vi "AlliGator Update Channel File Settings.vi"(8 "Error In":errorcluster, 9 "Channel Arithmetic":T1, 10 "Selected Channel Name":string, 11 "Available Channel Names":string[](array[string])) -> (0 "Error Out":errorcluster)   [LabVIEW 2021, in "AlliGator Settings.lvlib"]
doc: "Updates the values of the <B>Channel Name</b> and <B>Channel Arithmetic</b> controls, as well as of the hidden <B>Available Channel Names</b> indicator."
uses:
  AlliGator Settings.lvlib
  AlliGator Gate Arithmetic.ctl
  AlliGator Settings Event.ctl
  AlliGator Settings Window Messages.ctl
  AlliGator Dual-Channel Datasets.lvlib
panel:
  # "see the AlliGator License on the block diagram (Ctrl+E or Window:Show Block Diagram)"
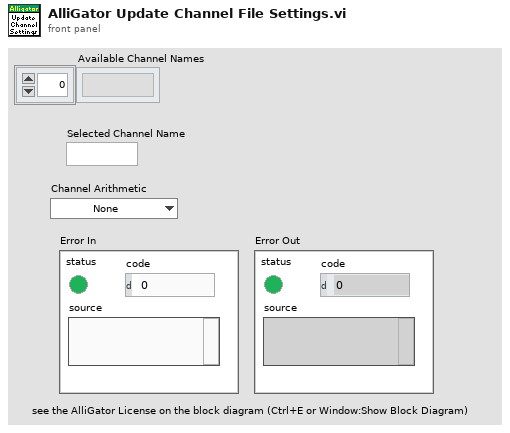
[diagram p1: front panel]
types:
  T1 = typedef "AlliGator Settings.lvlib/AlliGator Gate Arithmetic.ctl" = enum16{"None", "INT-G2", "G2/INT*<INT>", "(1 - G2/INT)*<INT>"}
  T2 = typedef "AlliGator Settings.lvlib/AlliGator Settings Event.ctl" = cluster{"AlliGator Settings Message":T3, "Sender":string, "Control Label":string, "Data":variant}
  T3 = typedef "AlliGator Settings.lvlib/AlliGator Settings Window Messages.ctl" = enum16{"Idle", "Subscribe", "Unsubscribe", "Refresh Parameter", "Refresh All Parameters", "Quit"}
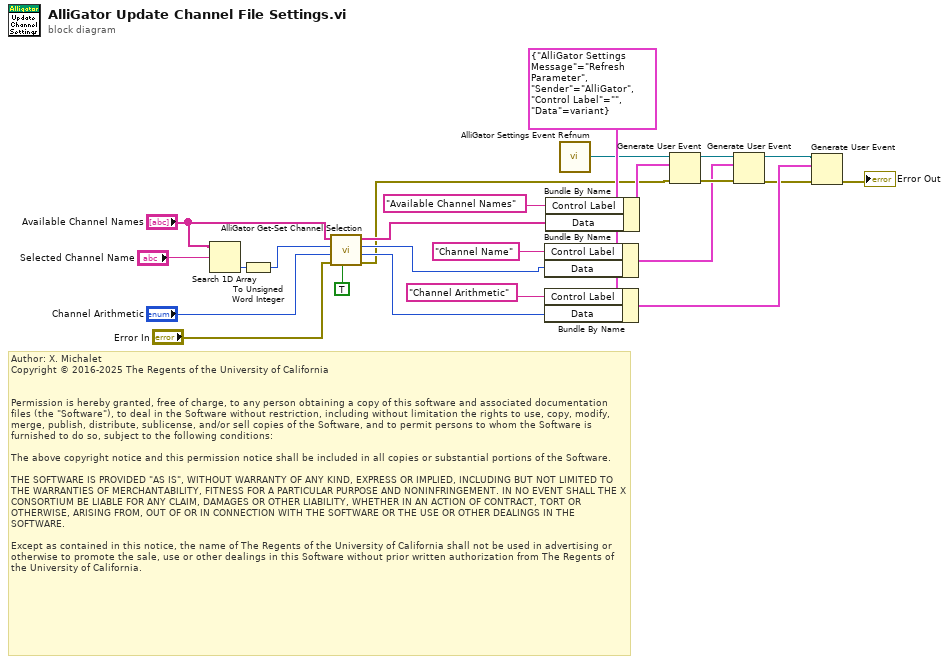
[diagram p0: block diagram]
diagram:
  w18 = T2 {"AlliGator Settings Message"=enum."Refresh Parameter", "Sender"="AlliGator", "Control Label"="", "Data"=variant} ("event data")
  # "Author: X. Michalet\nCopyright © 2016-2025 The Regents of the University of California\n \n\nPermission is hereby granted, free of charge, to any person obtaining a copy of this software and associated documentation files (the \"Software\"), to deal in the Software without restriction, including without limitation the rights to use, copy, modify, merge, publish, distribute, sublicense, and/or sell copies of the Software, and to permit persons to whom the Software is furnished to do so, subject to the following conditions:\n\nThe above copyright notice and this permission notice shall be included in all copies or substantial portions of the Software.\n\nTHE SOFTWARE IS PROVIDED \"AS IS\", WITHOUT WARRANTY OF ANY KIND, EXPRESS OR IMPLIED, INCLUDING BUT NOT LIMITED TO THE WARRANTIES OF MERCHANTABILITY, FITNESS FOR A PARTICULAR PURPOSE AND NONINFRINGEMENT. IN NO EVENT SHALL THE X CONSORTIUM BE LIABLE FOR ANY CLAIM, DAMAGES OR OTHER LIABILITY, WHETHER IN AN ACTION OF CONTRACT, TORT OR OTHERWISE, ARISING FROM, OUT OF OR IN CONNECTION WITH THE SOFTWARE OR THE USE OR OTHER DEALINGS IN THE SOFTWARE.\n\nExcept as contained in this notice, the name of The Regents of the University of California shall not be used in advertising or otherwise to promote the sale, use or other dealings in this Software without prior written authorization from The Regents of the University of California."
  n1 = Search 1D Array(1D array="Available Channel Names", element="Selected Channel Name") -> (index of element=w9:i32)  [unwired: 1 in]
  n2 = To Unsigned Word Integer(number=w9) -> (unsigned 16bit integer=w6:u16)
  n3 = call "AlliGator Get-Set Channel Selection.vi"("Set (T)/Get (F)"=TRUE, "error in (no error)"="Error In", "Channel Arithmetic"="Channel Arithmetic", "Selected Channel Name"=w6, "Available Channel Names"="Available Channel Names") -> ("error out"=w2:errorcluster, "Channel Arithmetic"=w3:T1, "Selected Channel Name"=w5:u16, "Available Channel Names"=w7:string[])  [unwired: 3 in]
  n4 = Bundle By Name(cluster=w18, "Control Label"="Channel Name", "Data"=w5) -> (w16:T2)
  n5 = Bundle By Name(cluster=w18, "Control Label"="Channel Arithmetic", "Data"=w3) -> (w21:T2)
  n6 = Bundle By Name(cluster=w18, "Control Label"="Available Channel Names", "Data"=w7) -> (w14:T2)
  n7 = call "AlliGator Settings Event Refnum.vi"() -> ("AlliGator Settings Event Refnum"=w13:refnum<user-event>)  [unwired: 8 in, 1 out]
  n8 = Generate User Event(user event=w13, event data cluster=w14, error in=w2) -> (user event out=w15:refnum<user-event>, error out=w17:errorcluster)  [unwired: 1 in]
  n9 = Generate User Event(user event=w15, event data cluster=w16, error in=w17) -> (user event out=w19:refnum<user-event>, error out=w20:errorcluster)  [unwired: 1 in]
  n10 = Generate User Event(user event=w19, event data cluster=w21, error in=w20) -> (error out=→"Error Out":errorcluster)  [unwired: 1 in, 1 out]
